vi "comm open2.vi"(4 "error in (no error)":errorcluster, 6 "open duplicate?":bool, 7 "Comm Port Name":string) -> (0 "error out":errorcluster, 1 "created new?":bool, 3 "Comm Handle":u32)   [LabVIEW 2017, in "lvserial.lvlib"]
doc: "Opens the serial port. If the duplicate value is true, only a duplicate of the serial port will be opened (if the serial port is already open)."
uses:
  lvserial.lvlib
  lvserial.dll
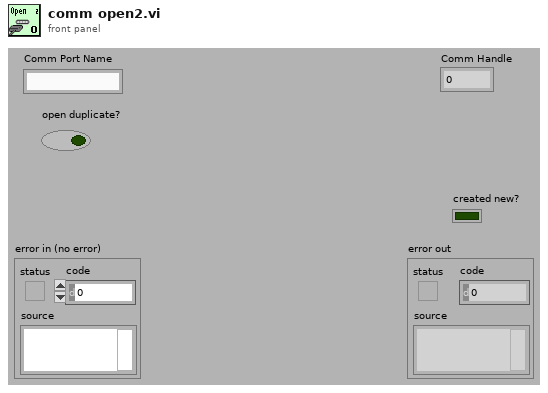
[diagram p1: front panel]
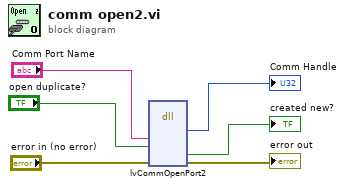
[diagram p0: block diagram]
diagram:
  n1 = dll-call lib="lvserial.dll" fn="lvCommOpenPort2"("port"="Comm Port Name", "open duplicate?"="open duplicate?", "error in (no error)"="error in (no error)") -> ("phComm"=→"Comm Handle":u32, "created new?"=→"created new?":bool, "error in (no error)"=→"error out":errorcluster)  [unwired: 5 in, 5 out]
